vi "McCamyCCT.vi"(10 "y":dbl, 11 "x":dbl) -> (3 "CCT":dbl)   [LabVIEW 2011]
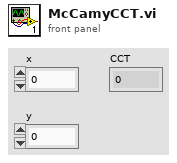
[diagram p1: front panel]
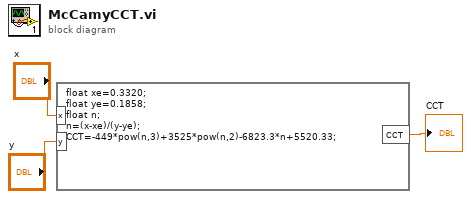
[diagram p0: block diagram]
diagram:
  n1 = formula code="float xe=0.3320;\nfloat ye=0.1858;\nfloat n;\nn=(x-xe)/(y-ye);\nCCT=-449*pow(n,3)+3525*pow(n,2)-6823.3*n+5520.33;"("x"="x", "y"="y") -> ("CCT"=→"CCT":dbl)
